vi "GET File Content.vi"(8 "错误输入":errorcluster, 9 "文件源":enum16{"本地", "Redis"}(ring), 10 "Redis TCP引用":refnum<k5>, 11 "File Path":path) -> (0 "错误输出":errorcluster, 2 "gzip":bool, 3 "File Content":string)   [LabVIEW 2019, in "HTTP Server.lvlib"]
uses:
  HTTP Server.lvlib
  REDIS/Palette/Redis Commands/Hashes/HGET.vi
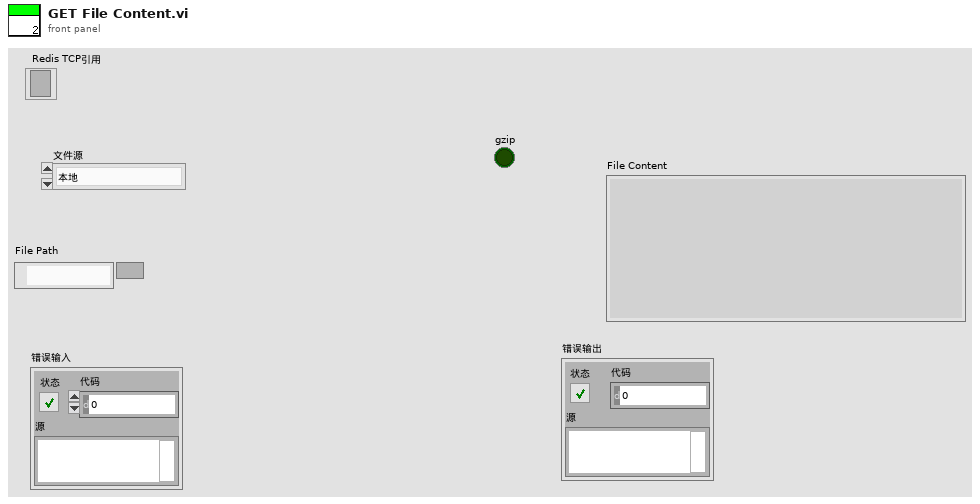
[diagram p1: front panel]
types:
  T1 = typedef "redis-data.ctl" = cluster{"type":enum16{"None", "Error", "Status", "Nil", "Integer", "String", "Multibulk"}, "integer":i64, "string":string, "multibulk":variant[], "string data":string[]}
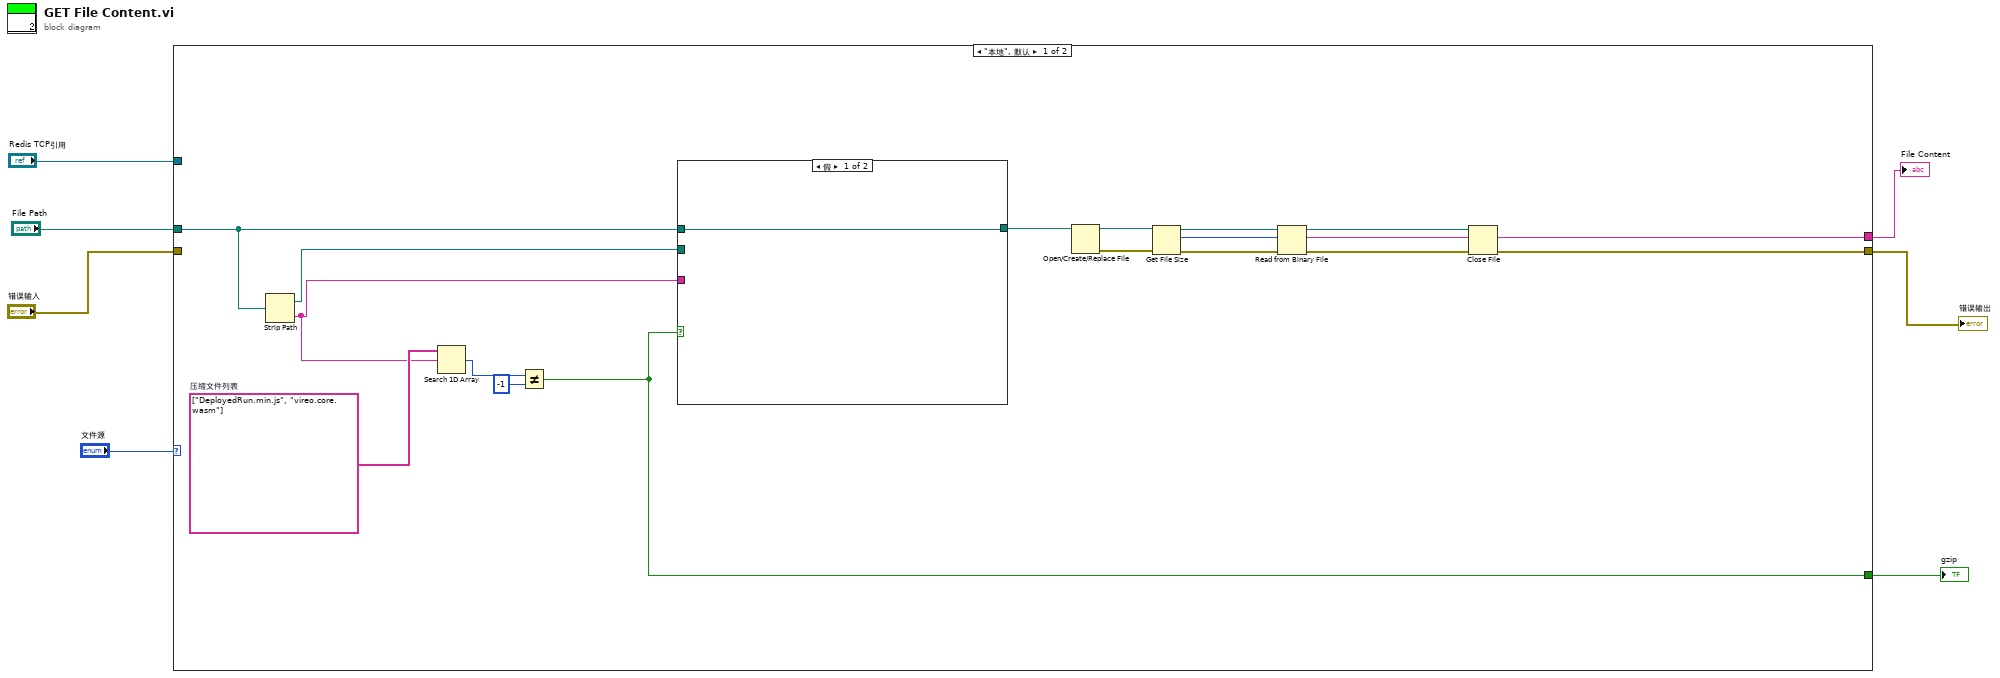
[diagram p0: block diagram]
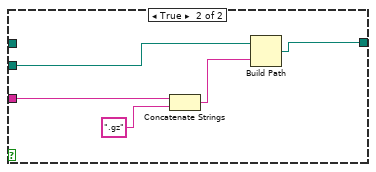
[diagram p2: hidden frame]
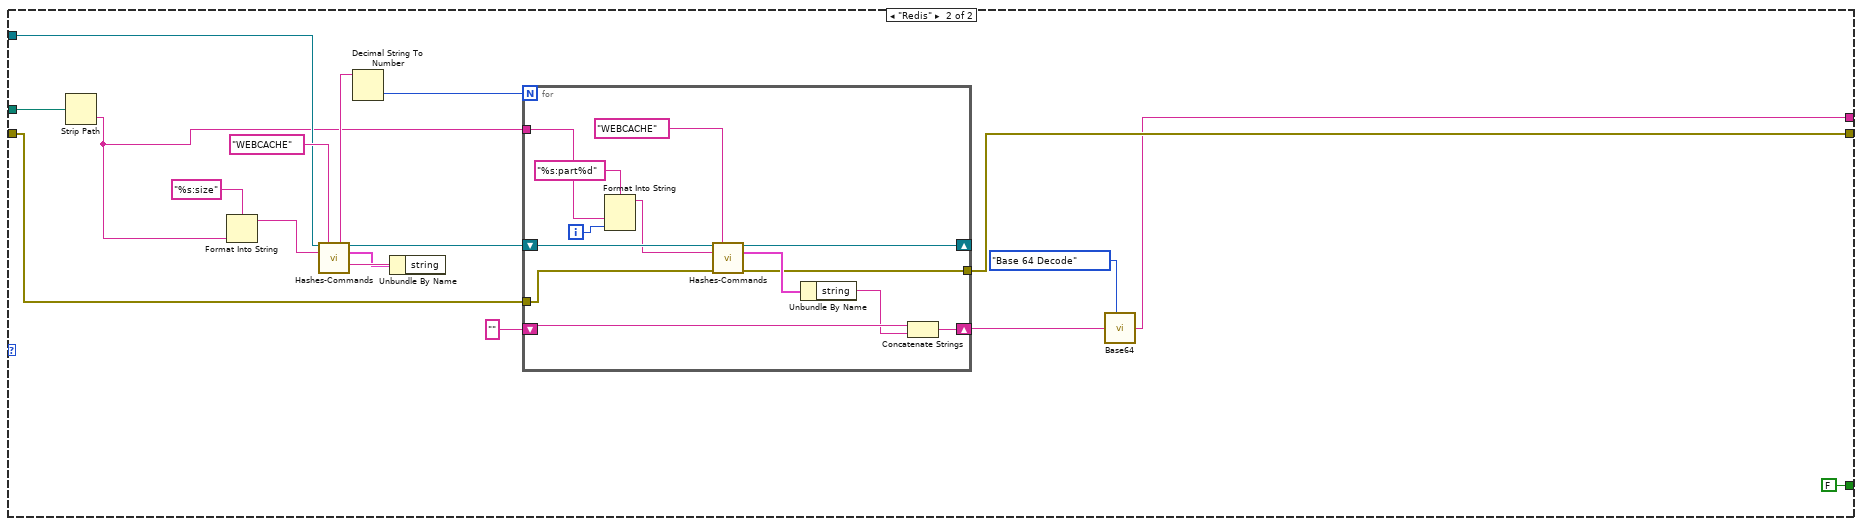
[diagram p3: hidden frame]
diagram:
  n1 = case shown="\"本地\", 默认" "文件源" {
    tunnel: "File Path" -> [w15 w40]
    tunnel: "错误输入" -> [_ w37]
    tunnel: [w24 w36] -> w5
    tunnel: [w21 w33] -> w4
    tunnel: "Redis TCP引用" -> [_ w35]
    tunnel: [w9 FALSE] -> w1
    frame "本地", Default {
      w12 = string[] ["DeployedRun.min.js", "vireo.core.wasm"]  # 压缩文件列表
      n2 = Strip Path(path=w15) -> (stripped path=w13:path, name=w8:string)
      n3 = Search 1D Array(1D array=w12, element=w8) -> (index of element=w11:i32)  [unwired: 1 in]
      n4 = Not Equal?(x=w11, y=-1) -> (x != y?=w9:bool)
      n5 = case shown="假" w9 {
        tunnel: w15 -> [w25 _]
        tunnel: [w25 w30] -> w14
        tunnel: w13 -> [_ w29]
        tunnel: w8 -> [_ w27]
        frame False {
        }
        frame True {
          n6 = Concatenate Strings(w27, ".gz" ("y")) -> (w26:string)
          n7 = Build Path(base path=w29, name or relative path=w26) -> (appended path=w30:path)
        }
      }
      n8 = Open/Create/Replace File(file path (use dialog)=w14) -> (refnum out=w20:refnum<file>, error out=w19:errorcluster)  [unwired: 5 in, 1 out]
      n9 = Get File Size(file=w20, error in=w19) -> (refnum out=w18:refnum<file>, size (in bytes)=w16:i64, 0:w17:errorcluster)
      n10 = Read from Binary File(8:w17, 10:w16, 11:w18) -> (0:w23:errorcluster, 2:w21:string, 3:w22:refnum<file>)  [unwired: 3 in, 1 out]
      n11 = Close File(refnum=w22, error in=w23) -> (error out=w24:errorcluster)  [unwired: 1 out]
    }
    frame "Redis" {
      n12 = Strip Path(path=w40) -> (name=w34:string)  [unwired: 1 out]
      n13 = Format Into String(format string="%s:size" ("Field"), w34) -> (resulting string=w38:string)  [unwired: 2 in, 1 out]
      n14 = call-poly "Hashes-Commands.vi"("redis连接ID"=w35, "Key"="WEBCACHE", "Field"=w38) -> ("redis连接ID"=w45:refnum<k5>, "Data"=w46:T1)  [unwired: 10 in, 1 out]
      n15 = Unbundle By Name(w46) -> ("string"=w47:string)
      n16 = Decimal String To Number(string=w47) -> (number=w32:i32)  [unwired: 2 in, 1 out]
      n17 = for {
        N: w32 -> [_]
        shift-right: [w56] -> _
        shift-left: w45 -> [w60]
        shift-right: [w52] -> w44
        shift-left: "" -> [w54]
        tunnel: w34 -> [w50]
        tunnel: w37 -> [w49]
        tunnel: [w48] -> w36
        i -> [w51]
        n18 = Format Into String(format string="%s:part%d" ("Key"), w50, w51) -> (resulting string=w57:string)  [unwired: 2 in, 1 out]
        n19 = call-poly "Hashes-Commands.vi"("redis连接ID"=w60, "Key"="WEBCACHE", "Field"=w57, "error in"=w49) -> ("redis连接ID"=w56:refnum<k5>, "Data"=w55:T1, "error out"=w48:errorcluster)  [unwired: 9 in]
        n20 = Unbundle By Name(w55) -> ("string"=w53:string)
        n21 = Concatenate Strings(w54, w53) -> (w52:string)
      }
      n22 = call "Base64.vi"("Switch"=enum16{"Base 64 Encode", "Base 64 Decode"}."Base 64 Decode", "Input String"=w44) -> ("Output String"=w33:string)  [unwired: 5 in]
    }
  }
  "错误输出" <- w5
  "File Content" <- w4
  "gzip" <- w1
